vi "Test 1.vi"() -> ()   [LabVIEW 2013]
uses:
  Reload Pro/Reload-pro.lvclass
panel:
  out "Setpoint Out":dbl
  in  "stop":bool
  in  "Horizontal Pointer Slide":dbl
  in  "VISA resource name":refnum<visa-resource-name>
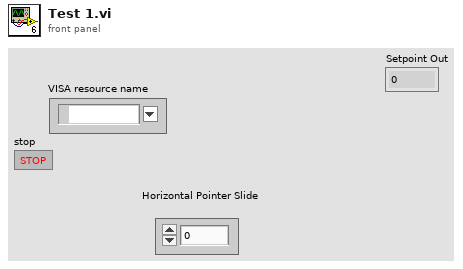
[diagram p1: front panel]
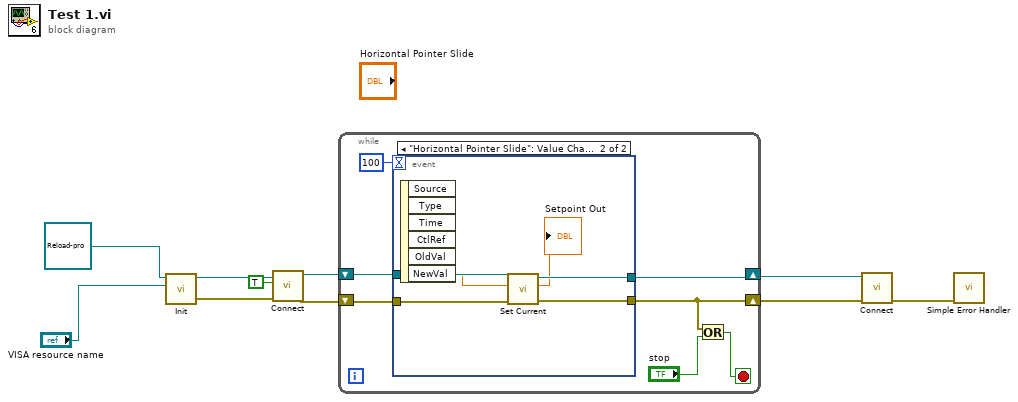
[diagram p0: block diagram]
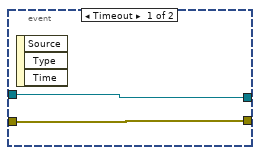
[diagram p2: hidden frame]
diagram:
  n1 = call-dynamic "Init.vi"("VISA resource name"="VISA resource name", "Reload-pro in"=refnum<class "Reload-pro.lvclass"> refnum ("Reload-pro.lvclass")) -> ("error out"=w7:errorcluster, "Reload-pro out"=w8:refnum<class "Reload-pro.lvclass">)  [unwired: 8 in]
  n2 = call-dynamic "Connect.vi"("error in (no error)"=w7, "Connect?"=TRUE, "Reload-pro in"=w8) -> ("error out"=w1:errorcluster, "Reload-pro out"=w4:refnum<class "Reload-pro.lvclass">)  [unwired: 7 in]
  n3 = while {
    shift-right: [w16] -> w3
    shift-left: w4 -> [w17]
    shift-right: [w13] -> w2
    shift-left: w1 -> [w15]
    stop <- w11 stop-if-true
    n4 = event shown="[1] \"Horizontal Pointer Slide\": Value Change" {
      selector: _ -> [_ _]
      dyn-events: _ -> [_ _]
      timeout: 100 -> [_ _]
      tunnel: w17 -> [w19 w25]
      tunnel: [w19 w24] -> w16
      tunnel: [w18 w23] -> w13
      tunnel: w15 -> [w18 w22]
      event Timeout {
        n5 = event-data() -> ()  [unwired: 1 in, 3 out]
      }
      event "Horizontal Pointer Slide": Value Change {
        n6 = event-data() -> ("NewVal"=w21:dbl)  [unwired: 1 in, 5 out]
        n7 = call-dynamic "Set Current.vi"("error in (no error)"=w22, "Setpoint In"=w21, "Reload-pro in"=w25) -> ("error out"=w23:errorcluster, "Setpoint Out"=→"Setpoint Out":dbl, "Reload-pro out"=w24:refnum<class "Reload-pro.lvclass">)  [unwired: 6 in]
      }
    }
    n8 = Or(x=w13, y="stop") -> (x .or. y?=w11:bool)
  }
  n9 = call-dynamic "Connect.vi"("error in (no error)"=w2, "Reload-pro in"=w3) -> ("error out"=w5:errorcluster)  [unwired: 8 in, 1 out]
  n10 = call <vilib>:"Simple Error Handler.vi"("error in (no error)"=w5) -> ()  [unwired: 4 in, 5 out]
